vi "RIO_Formula Node.vi"(0 "X":string, 1 "Y":string, 3 "URAPI Script":T1={"Script"="", "Whiles"=[], "Ifs"=[], "Supress Err"=TRUE, "Errors"=""}, 4 "formula":string="x+y") -> (2 "Z":string, 5 "URAPI Script Out":T1={"Script"="", "Whiles"=[], "Ifs"=[], "Supress Err"=TRUE, "Errors"=""})   [LabVIEW 2012]
doc: "Calculates the formula specified in the formula input. Supports the functions: SIN(x), COS(x), TAN(x), ASIN(x), ACOS(x), ATAN(x), LN(x), EXP(x), LOG(x), ABS(x), SQRT(x), SGN(x). The calculator is not case sensitive. \n\n<B>Inputs\nformula </B> is a string containing the formula to be evaluated.\n<B>X </B> is a number represented by the variable X in the formula. \n<B>Y </B> is a number represented by the variable y in the formula. \n<B>NXT </B> connects to NXT terminal of previous VI to establish the flow of the program.\n\n<B>Outputs\nZ </B> is the calculated result number represented by the variable z in the formula. \n<B>NXT</B> wires to NXT terminal of next VI to establish the flow of the program.\n<B>operation stack</B>"
uses:
  <userlib>/BotSpeak/VIs/Direct/URAPI_Control.ctl
panel:
  out "Stack out":string[](array[string])
  out "operation stack":string[](array[string])
  # "SIN(x)\nCOS(x)\nTAN(x)\nATAN(x)\nLN(x)\nEXP(x)\nLOG(x)\nABS(x)\nSQRT(x)\nSGN(x)"
  # "This supports:\n^+-*/%\n&| (bitwise)"
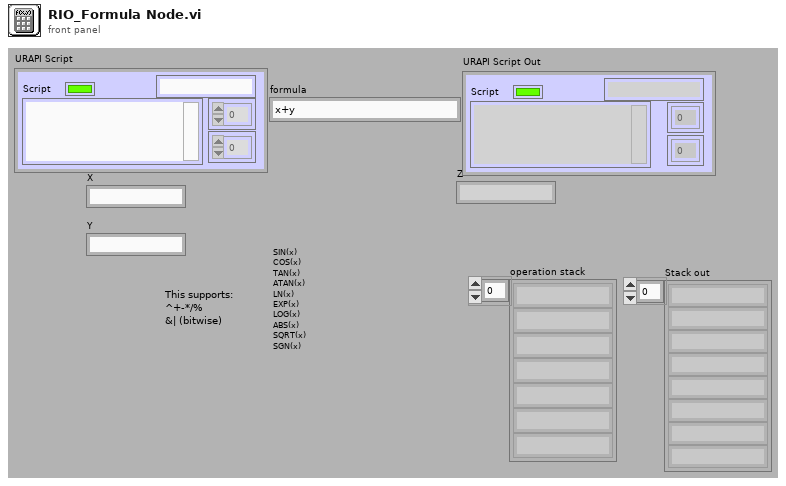
[diagram p1: front panel]
types:
  T1 = typedef "URAPI_Control.ctl" = cluster{"Script":string, "Whiles":u8[], "Ifs":u8[], "Supress Err":bool, "Errors":string}
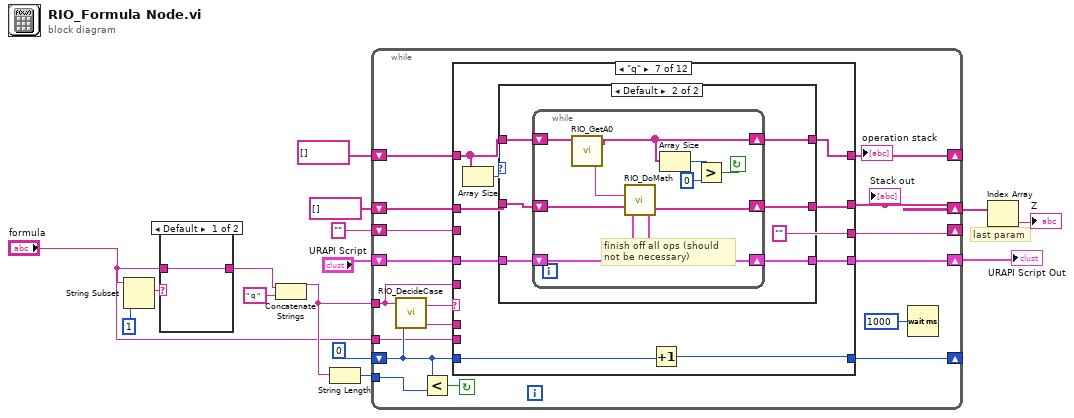
[diagram p0: block diagram]
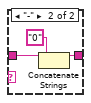
[diagram p2: hidden frame]
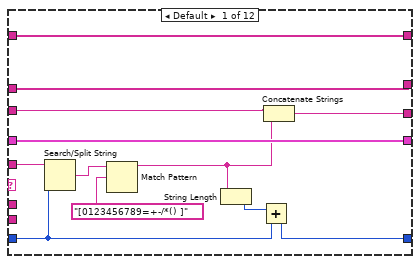
[diagram p3: hidden frame]
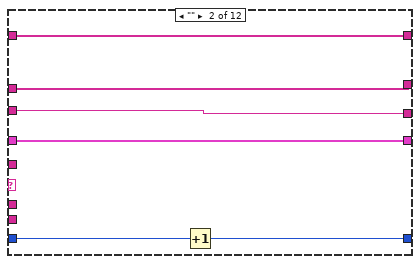
[diagram p4: hidden frame]
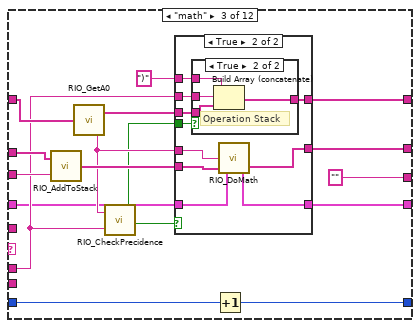
[diagram p5: hidden frame]
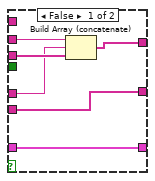
[diagram p6: hidden frame]
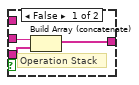
[diagram p7: hidden frame]
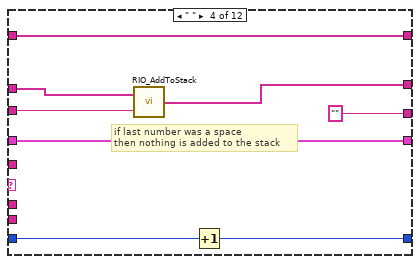
[diagram p8: hidden frame]
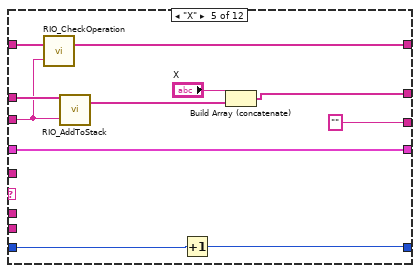
[diagram p9: hidden frame]
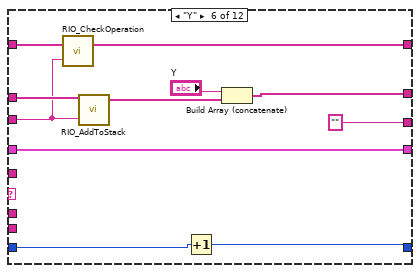
[diagram p10: hidden frame]
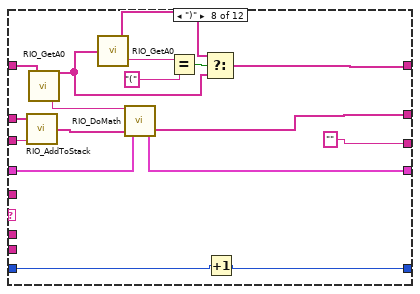
[diagram p12: hidden frame]
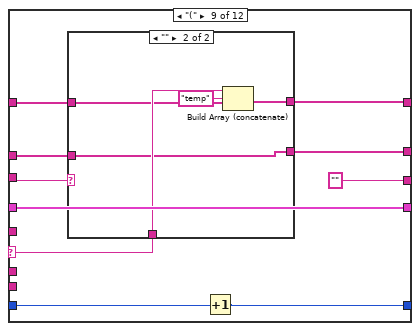
[diagram p13: hidden frame]
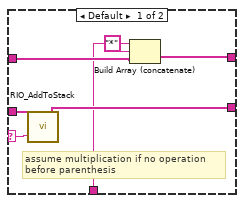
[diagram p14: hidden frame]
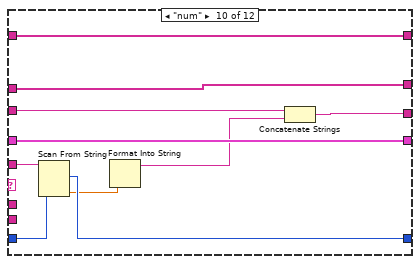
[diagram p15: hidden frame]
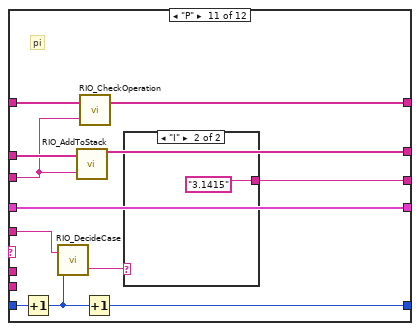
[diagram p16: hidden frame]
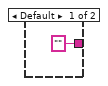
[diagram p17: hidden frame]
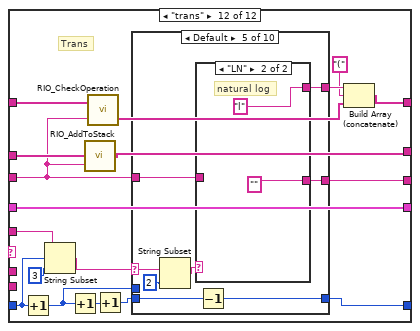
[diagram p18: hidden frame]
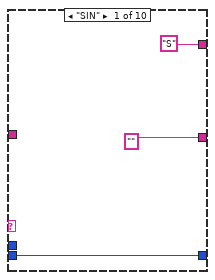
[diagram p19: hidden frame]
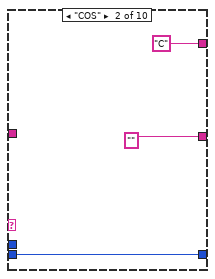
[diagram p20: hidden frame]
diagram:
  # "last param"
  n1 = String Subset(string="formula", length (rest)=1 ("length (rest)")) -> (substring=w3:string)  [unwired: 1 out]
  n2 = case shown="Default" w3 {
    tunnel: [w16 w19] -> w2
    tunnel: "formula" -> [w16 w18]
    frame Default {
    }
    frame "-" {
      n3 = Concatenate Strings("0" ("string"), w18) -> (w19:string)
    }
  }
  n4 = Concatenate Strings(w2, " q " ("string")) -> (w9:string)
  n5 = String Length(string=w9) -> (length=w10:i32)
  n6 = while {
    tunnel: w10 -> [w36]
    shift-right: [w30] -> w11
    shift-left: string[] [] ("Stack") -> [w33]
    shift-right: [w31] -> _
    shift-left: "" -> [w34]
    shift-right: [w29] -> _
    shift-left: string[] [] ("Stack") -> [w32]
    tunnel: w9 -> [w25]
    shift-right: [w24] -> _
    shift-left: 0 -> [w26]
    shift-right: [w22] -> w5
    shift-left: "URAPI Script" -> [w23]
    tunnel: "formula" -> [w21]
    stop <- w35 continue-if-true
    n7 = call <userlib>:"RIO_DecideCase.vi"("i"=w26, "string"=w25) -> ("symbol"=w27:string, "case"=w28:string)
    n8 = Less?(x=w26, y=w36) -> (x < y?=w35:bool)
    n9 = case shown="\"q\"" w28 {
      selector: w28 -> [_ _ _ _ _ _ _ _ w179 _ _ _]
      tunnel: w34 -> [w44 w54 w69 w100 w104 w117 _ w169 w174 w202 w203 w230]
      tunnel: [w43 w54 "" "" "" "" "" "" "" w201 w209 w234] -> w31
      tunnel: w33 -> [w48 w53 w70 w101 w105 w118 w131 w168 w173 w200 w207 w231]
      tunnel: [w48 w53 w66 w99 w111 w123 w130 w166 w172 w200 w206 w229] -> w30
      tunnel: w32 -> [w47 w52 w64 w98 w107 w115 w125 w165 w178 w199 w205 w228]
      tunnel: [w47 w52 w68 w98 w106 w114 w129 w158 w177 w199 w204 w217] -> w29
      tunnel: w27 -> [_ _ w61 _ _ _ _ _ _ _ _ _]
      tunnel: [w40 w50 w62 w96 w109 w120 w132 w156 w175 w195 w212 w227] -> w24
      tunnel: w26 -> [w38 w51 w63 w97 w110 w121 w133 w157 w176 w196 w214 w223]
      tunnel: w25 -> [w39 _ _ _ _ _ _ _ _ w197 w213 w224]
      tunnel: w23 -> [w46 w49 w56 w95 w108 w119 w128 w155 w171 w198 w208 w233]
      tunnel: [w46 w49 w55 w95 w108 w119 w127 w154 w171 w198 w208 w233] -> w22
      tunnel: w21 -> [_ _ _ _ _ _ _ _ _ _ _ _]
      frame Default {
        n10 = Search/Split String(string=w39, offset (0)=w38) -> (match + rest of string=w37:string)  [unwired: 1 in, 2 out]
        n11 = Match Pattern(string=w37, regular expression="[0123456789=+-/*() ]") -> (before substring=w42:string)  [unwired: 1 in, 3 out]
        n12 = String Length(string=w42) -> (length=w41:i32)
        n13 = Add(x=w41, y=w38) -> (x+y=w40:u32)
        n14 = Concatenate Strings(w44, w42) -> (w43:string)
      }
      frame "" {
        n15 = Increment(x=w51) -> (x+1=w50:u32)
      }
      frame "math" {
        n16 = call <userlib>:"RIO_AddToStack.vi"("Number"=w69, "Stack in"=w70) -> ("Stack out"=w67:string[])
        n17 = call <userlib>:"RIO_GetA0.vi"("A[0..n]"=w64) -> ("A[1..n]"=w65:string[], "A[0]"=w59:string)
        n18 = call <userlib>:"RIO_CheckPrecidence.vi"("new op"=w61, "last op"=w59) -> ("lower precidence?"=w60:bool, "transidental end?"=w58:bool)
        n19 = case shown="True" w60 {
          tunnel: [w74 w87] -> w68
          tunnel: w61 -> [w75 w86]
          tunnel: w65 -> [w77 w85]
          tunnel: w59 -> [w76 w84]
          tunnel: w67 -> [w73 w83]
          tunnel: [w73 w82] -> w66
          tunnel: w58 -> [_ w81]
          tunnel: ")" -> [_ w80]
          tunnel: w56 -> [w72 w79]
          tunnel: [w72 w78] -> w55
          frame False {
            n20 = Build Array (concatenate)(w75, w76, w77) -> (w74:string[])
          }
          frame True {
            n21 = case shown="True" w81 {
              tunnel: [w90 w94] -> w87
              tunnel: w86 -> [w89 w91]
              tunnel: w85 -> [w88 w93]
              tunnel: w80 -> [_ w92]
              frame False {
                # "Operation Stack"
                n22 = Build Array (concatenate)(w89, w88) -> (w90:string[])
              }
              frame True {
                # "Operation Stack"
                n23 = Build Array (concatenate)(w92, w91, w93) -> (w94:string[])
              }
            }
            n24 = call <userlib>:"RIO_DoMath.vi"("Stack in"=w83, "Last Operation"=w84, "URAPI Script"=w79) -> ("Stack out"=w82:string[], "URAPI Script Out"=w78:T1)
          }
        }
        n25 = Increment(x=w63) -> (x+1=w62:u32)
      }
      frame " " {
        # "if last number was a space\nthen nothing is added to the stack"
        n26 = call <userlib>:"RIO_AddToStack.vi"("Number"=w100, "Stack in"=w101) -> ("Stack out"=w99:string[])
        n27 = Increment(x=w97) -> (x+1=w96:u32)
      }
      frame "X" {
        n28 = call <userlib>:"RIO_CheckOperation.vi"("String"=w104, "Stack in"=w107) -> ("Stack out"=w106:string[])
        n29 = call <userlib>:"RIO_AddToStack.vi"("Number"=w104, "Stack in"=w105) -> ("Stack out"=w103:string[])
        n30 = Increment(x=w110) -> (x+1=w109:u32)
        n31 = Build Array (concatenate)("X", w103) -> (w111:string[])
      }
      frame "Y" {
        n32 = call <userlib>:"RIO_CheckOperation.vi"("String"=w117, "Stack in"=w115) -> ("Stack out"=w114:string[])
        n33 = call <userlib>:"RIO_AddToStack.vi"("Number"=w117, "Stack in"=w118) -> ("Stack out"=w116:string[])
        n34 = Increment(x=w121) -> (x+1=w120:u32)
        n35 = Build Array (concatenate)("Y", w116) -> (w123:string[])
      }
      frame "q" {
        n36 = Array Size(array=w125) -> (size(s)=w126:i32)
        n37 = case shown="Default" w126 {
          tunnel: [w137 w143] -> w129
          tunnel: w131 -> [w136 w142]
          tunnel: [w136 w141] -> w130
          tunnel: w125 -> [w137 w140]
          tunnel: w128 -> [w135 w139]
          tunnel: [w135 w138] -> w127
          frame 0 {
          }
          frame Default {
            n38 = while {
              shift-right: [w153] -> w141
              shift-left: w142 -> [w152]
              shift-right: [w150] -> w143
              shift-left: w140 -> [w151]
              shift-right: [w144] -> w138
              shift-left: w139 -> [w145]
              stop <- w146 continue-if-true
              # "finish off all ops (should\nnot be necessary)"
              n39 = call <userlib>:"RIO_GetA0.vi"("A[0..n]"=w151) -> ("A[1..n]"=w150:string[], "A[0]"=w149:string)
              n40 = call <userlib>:"RIO_DoMath.vi"("Stack in"=w152, "Last Operation"=w149, "URAPI Script"=w145) -> ("Stack out"=w153:string[], "URAPI Script Out"=w144:T1)
              n41 = Array Size(array=w150) -> (size(s)=w148:i32)
              n42 = Greater?(x=w148, y=0) -> (0:w146:bool)
            }
          }
        }
        n43 = Increment(x=w133) -> (x+1=w132:u32)
      }
      frame ")" {
        n44 = call <userlib>:"RIO_AddToStack.vi"("Number"=w169, "Stack in"=w168) -> ("Stack out"=w167:string[])
        n45 = call <userlib>:"RIO_GetA0.vi"("A[0..n]"=w165) -> ("A[1..n]"=w159:string[], "A[0]"=w164:string)
        n46 = call <userlib>:"RIO_GetA0.vi"("A[0..n]"=w159) -> ("A[1..n]"=w160:string[], "A[0]"=w163:string)
        n47 = call <userlib>:"RIO_DoMath.vi"("Stack in"=w167, "Last Operation"=w164, "URAPI Script"=w155) -> ("Stack out"=w166:string[], "URAPI Script Out"=w154:T1)
        n48 = Equal?(x=w163, y="(") -> (x = y?=w161:bool)
        n49 = Select(t=w160, s=w161, f=w159) -> (s? t:f=w158:string[])
        n50 = Increment(x=w157) -> (x+1=w156:u32)
      }
      frame "(" {
        n51 = case shown="\"\"" w174 {
          selector: w174 -> [w184 _]
          tunnel: w179 -> [w182 w192]
          tunnel: w178 -> [w187 w191]
          tunnel: [w186 w190] -> w177
          tunnel: w173 -> [w185 w189]
          tunnel: [w183 w189] -> w172
          frame Default {
            # "assume multiplication if no operation\nbefore parenthesis"
            n52 = call <userlib>:"RIO_AddToStack.vi"("Number"=w184, "Stack in"=w185) -> ("Stack out"=w183:string[])
            n53 = Build Array (concatenate)(w182, "*" ("element"), w187) -> (w186:string[])
          }
          frame "" {
            n54 = Build Array (concatenate)(w192, "temp" ("element"), w191) -> (w190:string[])
          }
        }
        n55 = Increment(x=w176) -> (x+1=w175:u32)
      }
      frame "num" {
        n56 = Scan From String(input string=w197, initial scan location=w196) -> (offset past scan=w195:u32, output 1=w194:dbl)  [unwired: 3 in, 2 out]
        n57 = Format Into String(w194) -> (resulting string=w193:string)  [unwired: 3 in, 1 out]
        n58 = Concatenate Strings(w202, w193) -> (w201:string)
      }
      frame "P" {
        # "pi"
        n59 = Increment(x=w214) -> (x+1=w211:u32)
        n60 = call <userlib>:"RIO_DecideCase.vi"("i"=w211, "string"=w213) -> ("symbol"=w210:string)  [unwired: 1 out]
        n61 = call <userlib>:"RIO_AddToStack.vi"("Number"=w203, "Stack in"=w207) -> ("Stack out"=w206:string[])
        n62 = call <userlib>:"RIO_CheckOperation.vi"("String"=w203, "Stack in"=w205) -> ("Stack out"=w204:string[])
        n63 = Increment(x=w211) -> (x+1=w212:u32)
        n64 = case shown="\"I\"" w210 {
          tunnel: ["" "3.1415"] -> w209
          frame Default {
          }
          frame "I" {
          }
        }
      }
      frame "trans" {
        # "Trans"
        n65 = Increment(x=w223) -> (x+1=w225:u32)
        n66 = String Subset(string=w224, offset (0)=w223, length (rest)=3 ("length (rest)")) -> (substring=w221:string)
        n67 = Increment(x=w225) -> (x+1=w232:u32)
        n68 = call <userlib>:"RIO_AddToStack.vi"("Number"=w230, "Stack in"=w231) -> ("Stack out"=w229:string[])
        n69 = call <userlib>:"RIO_CheckOperation.vi"("String"=w230, "Stack in"=w228) -> ("Stack out"=w220:string[])
        n70 = Increment(x=w232) -> (x+1=w226:u32)
        n71 = case shown="Default" w221 {
          selector: w221 -> [_ _ _ _ w253 _ _ _ _ _]
          tunnel: ["" "" "" "" w255 "" "" "" "" ""] -> w234
          tunnel: w230 -> [_ _ _ _ w250 _ _ _ _ _]
          tunnel: [w236 w239 w242 w245 w249 w261 w264 w267 w270 w274] -> w227
          tunnel: w226 -> [w236 w239 w242 w246 w254 w261 w264 w267 w271 w274]
          tunnel: w225 -> [_ _ _ _ _ _ _ _ _ _]
          tunnel: ["S" "C" "T" "t" w248 "e" "L" "A" "R" "N"] -> w219
          frame "SIN" {
          }
          frame "COS" {
          }
          frame "TAN" {
          }
          frame "ATA" {
            # "atan"
            n72 = Increment(x=w246) -> (x+1=w245:u32)
          }
          frame Default {
            n73 = String Subset(string=w253, length (rest)=2 ("length (rest)")) -> (substring=w252:string)  [unwired: 1 in]
            n74 = case shown="\"LN\"" w252 {
              tunnel: [w257 ""] -> w255
              tunnel: w250 -> [w257 _]
              tunnel: ["" "l"] -> w248
              frame Default {
              }
              frame "LN" {
                # "natural log"
              }
            }
            n75 = Decrement(x=w254) -> (x-1=w249:u32)
          }
          frame "EXP" {
            # "exp"
          }
          frame "LOG" {
            # "Log b 10"
          }
          frame "ABS" {
            # "ABS"
          }
          frame "SQR" {
            # "square root"
            n76 = Increment(x=w271) -> (x+1=w270:u32)
          }
          frame "SGN" {
            # "sign"
          }
        }
        n77 = Build Array (concatenate)(w219, "(", w220) -> (w217:string[])
      }
    }
    "operation stack" <- w29
    "Stack out" <- w30
    n78 = Wait (ms)(milliseconds to wait=u32 1000) -> ()  [unwired: 1 out]
  }
  "URAPI Script Out" <- w5
  n79 = Index Array(array=w11) -> (element=→"Z":string)  [unwired: 1 in]
